vi "UDPchecker_v1.vi"(10 "new string":string, 11 "old string":string) -> (3 "output string":string)   [LabVIEW 2016]
panel:
  # ">>>"
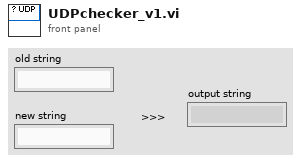
[diagram p1: front panel]
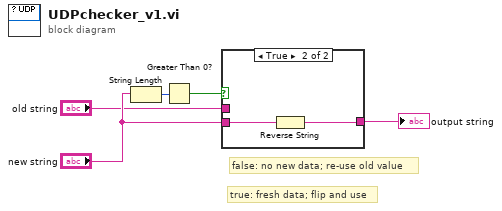
[diagram p0: block diagram]
diagram:
  # "true: fresh data; flip and use"
  # "false: no new data; re-use old value"
  n1 = String Length(string="new string") -> (length=w4:i32)
  n2 = Greater Than 0?(x=w4) -> (x > 0?=w3:bool)
  n3 = case shown="True" w3 {
    tunnel: "old string" -> [w6 _]
    tunnel: "new string" -> [_ w8]
    tunnel: [w6 w7] -> w2
    frame False {
    }
    frame True {
      n4 = Reverse String(1:w8) -> (0:w7:string)
    }
  }
  "output string" <- w2
